vi "Save Data File.vi"(0 "File Type":T1, 1 "Data":dbl[](array[numeric]), 2 "Open File Location":bool, 3 "error in (no error)":errorcluster) -> (10 "error out":errorcluster)   [LabVIEW 2020]
uses:
  controls/File Type.ctl
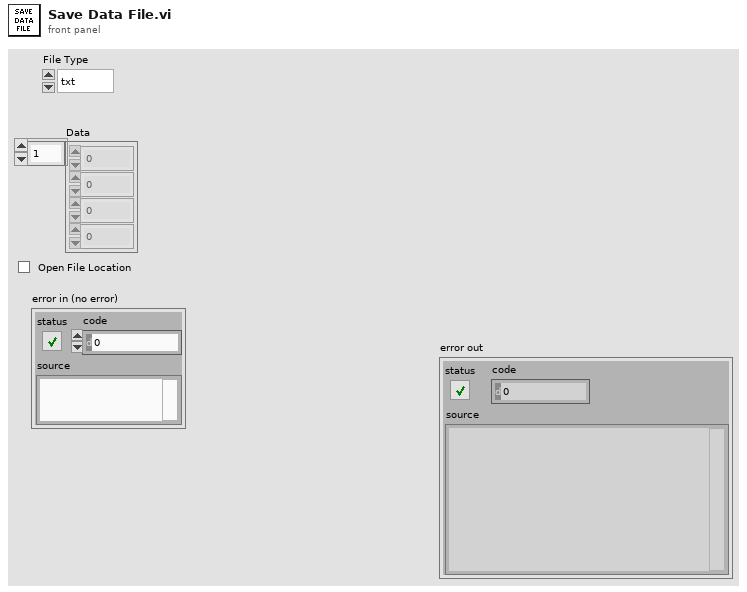
[diagram p1: front panel]
types:
  T1 = typedef "File Type.ctl" = enum16{"txt", "csv", "tdms", ""}
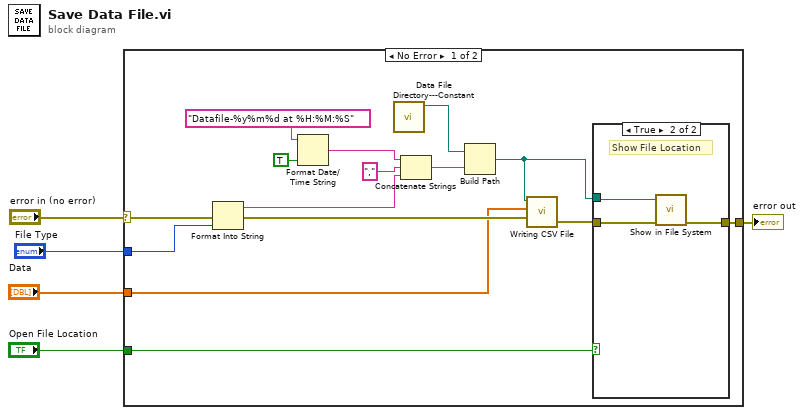
[diagram p0: block diagram]
diagram:
  n1 = case shown="No Error" "error in (no error)" {
    selector: "error in (no error)" -> [w14 _]
    tunnel: "File Type" -> [w16 _]
    tunnel: "Open File Location" -> [w13 _]
    tunnel: [w9 _] -> w3
    tunnel: "Data" -> [w7 _]
    frame No Error {
      n2 = Format Into String(error in=w14, w16) -> (resulting string=w15:string, error out=w11:errorcluster)  [unwired: 2 in]
      n3 = Format Date/Time String(time format string (%c)="Datafile-%y%m%d at %H:%M:%S", UTC format=TRUE) -> (date/time string=w19:string)  [unwired: 1 in]
      n4 = call "Data File Directory---Constant.vi"() -> ("Data File directory"=w12:path)  [unwired: 11 in]
      n5 = Concatenate Strings(w19, "," ("element"), w15) -> (w17:string)
      n6 = Build Path(base path=w12, name or relative path=w17) -> (appended path=w8:path)
      n7 = call "Writing CSV File.vi"("error in (no error)"=w11, "Data"=w7, "Path"=w8) -> ("error out"=w10:errorcluster)  [unwired: 8 in]
      n8 = case shown="True" w13 {
        tunnel: w10 -> [_ w22]
        tunnel: [_ w21] -> w9
        tunnel: w8 -> [_ w23]
        frame False {
        }
        frame True {
          # "Show File Location \n\n\n\nShow File Location"
          n9 = call <vilib>:"Show in File System.vi"("error in (no error)"=w22, "file or directory path"=w23) -> ("error out"=w21:errorcluster)  [unwired: 9 in]
        }
      }
    }
    frame Error {
    }
  }
  "error out" <- w3
